vi "Handshake.vi"(8 "error in (no error)":errorcluster, 10 "JQMHStartup in":refnum<class "RQMHStartup.lvclass">, 11 "JQMHModule in":refnum<class "RQMHModule.lvclass">) -> (0 "error out":errorcluster, 1 "HandshakeComplete?":bool, 3 "JQMHModule out":refnum<class "RQMHModule.lvclass">)   [LabVIEW 2024, in "RQMHModule.lvclass"]
uses:
  RQMHModule.lvclass
  Startup/RQMHStartup.lvclass
  RQMHModule.lvclass/RQMHModule.ctl
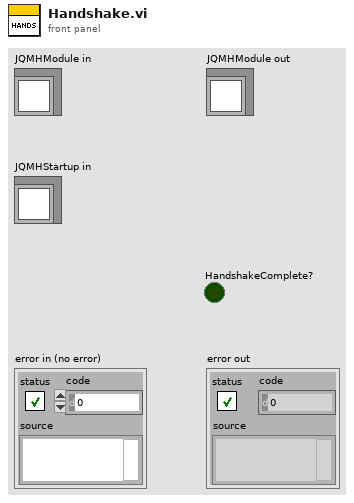
[diagram p1: front panel]
types:
  T1 = typedef "RQMHStartup.lvclass/Command.ctl" = enum16{"Default", "No Override", "Error", "ACK Created", "ACK Mod Reg", "ACK Caller Reg"}
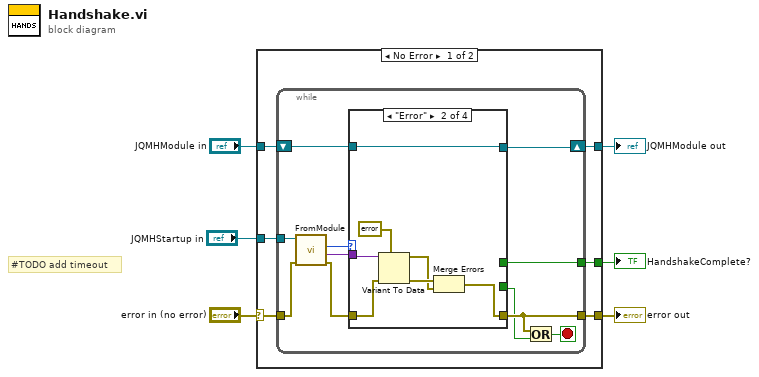
[diagram p0: block diagram]
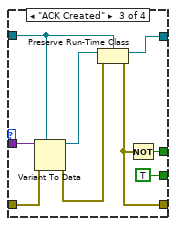
[diagram p3: hidden frame]
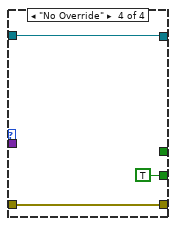
[diagram p4: hidden frame]
diagram:
  # "#TODO add timeout"
  n1 = case shown="No Error" "error in (no error)" {
    selector: "error in (no error)" -> [w7 w46]
    tunnel: "JQMHModule in" -> [w12 w45]
    tunnel: [w11 w45] -> w5
    tunnel: [w10 _] -> w4
    tunnel: "JQMHStartup in" -> [w9 _]
    tunnel: [w8 w46] -> w1
    frame No Error {
      n2 = while {
        tunnel: w7 -> [w21]
        shift-right: [w18] -> w11
        shift-left: w12 -> [w19]
        tunnel: [w17] -> w8
        tunnel: [w14] -> w10
        tunnel: w9 -> [w13]
        stop <- w16 stop-if-true
        n3 = call "FromModule.vi"("error in (no error)"=w21, "JQMHStartup in"=w13) -> ("error out"=w20:errorcluster, "Data"=w22:variant, "Command"=w23:T1)  [unwired: 6 in, 1 out]
        n4 = case shown="\"Error\"" w23 {
          tunnel: w22 -> [_ w32 w41 _]
          tunnel: w20 -> [w25 w31 w37 w43]
          tunnel: [w25 w28 w33 w43] -> w17
          tunnel: w19 -> [w24 w30 w40 w44]
          tunnel: [w24 w30 w38 w44] -> w18
          tunnel: [_ _ TRUE TRUE] -> w15
          tunnel: [_ _ w35 _] -> w14
          frame Default {
          }
          frame "Error" {
            n5 = Variant To Data(error in=w31, type=errorcluster {"status"=FALSE, "code"=0, "source"=""} ("error out"), Variant=w32) -> (data=w26:errorcluster, error out=w29:errorcluster)
            n6 = Merge Errors(w29, w26) -> (w28:errorcluster)
          }
          frame "ACK Created" {
            n7 = Variant To Data(error in=w37, type=w40, Variant=w41) -> (data=w39:refnum<class "RQMHModule.lvclass">, error out=w36:errorcluster)
            n8 = Preserve Run-Time Class(object in=w39, error in=w36, 2:w40) -> (object out=w38:refnum<class "RQMHModule.lvclass">, error out=w33:errorcluster)
            n9 = Not(x=w33) -> (.not. x?=w35:bool)
          }
          frame "No Override" {
          }
        }
        n10 = Or(x=w17, y=w15) -> (x .or. y?=w16:bool)
      }
    }
    frame Error {
    }
  }
  "error out" <- w1
  "JQMHModule out" <- w5
  "HandshakeComplete?" <- w4
